vi "ALLPROPS0dll.vi"(8 "error in (no error)":errorcluster, 11 "Inputs":T2) -> (0 "error out":errorcluster, 3 "Outputs":T1)   [LabVIEW 2021]
uses:
  REFPROP.dll
panel:
  # "REFPROP-ALLPROPS0dll.vi"
  # "void ALLPROPS0dll(int *iIn, int *iOut/* 200 */, int *iFlag, double *T, double *D, double *z/* 20 */, double *Output/* 200 */, int *ierr, char *herr, int herr_length/* 255 */);"
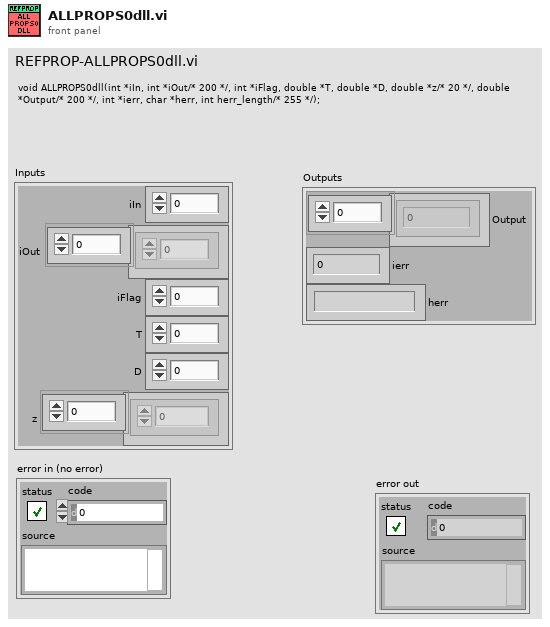
[diagram p1: front panel]
types:
  T1 = cluster{"Output":dbl[], "ierr":i32, "herr":string}
  T2 = cluster{"iIn":i32, "iOut":i32[], "iFlag":i32, "T":dbl, "D":dbl, "z":dbl[]}
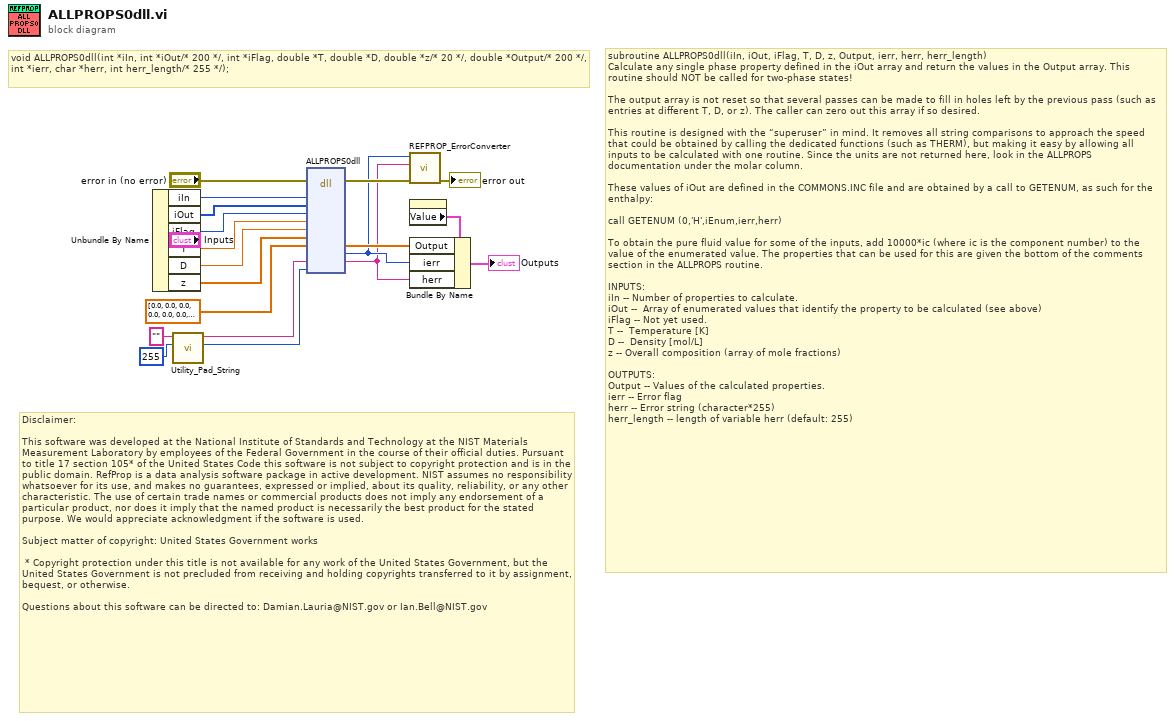
[diagram p0: block diagram]
diagram:
  # "void ALLPROPS0dll(int *iIn, int *iOut/* 200 */, int *iFlag, double *T, double *D, double *z/* 20 */, double *Output/* 200 */, int *ierr, char *herr, int herr_length/* 255 */);"
  # "Disclaimer:\n\nThis software was developed at the National Institute of Standards and Technology at the NIST Materials Measurement Laboratory by employees of the Federal Government in the course of their official duties. Pursuant to title 17 section 105* of the United States Code this software is not subject to copyright protection and is in the public domain. RefProp is a data analysis software package in active development. NIST assumes no responsibility whatsoever for its use, and makes no guarantees, expressed or implied, about its quality, reliability, or any other characteristic. The use of certain trade names or commercial products does not imply any endorsement of a particular product, nor does it imply that the named product is necessarily the best product for the stated purpose. We would appreciate acknowledgment if the software is used.\n \nSubject matter of copyright: United States Government works\n  \n * Copyright protection under this title is not available for any work of the United States Government, but the United States Government is not precluded from receiving and holding copyrights transferred to it by assignment, bequest, or otherwise.\n\nQuestions about this software can be directed to: Damian.Lauria@NIST.gov or Ian.Bell@NIST.gov"
  # "subroutine ALLPROPS0dll(iIn, iOut, iFlag, T, D, z, Output, ierr, herr, herr_length)\nCalculate any single phase property defined in the iOut array and return the values in the Output array. This routine should NOT be called for two-phase states!\n\nThe output array is not reset so that several passes can be made to fill in holes left by the previous pass (such as entries at different T, D, or z). The caller can zero out this array if so desired.\n\nThis routine is designed with the “superuser” in mind. It removes all string comparisons to approach the speed that could be obtained by calling the dedicated functions (such as THERM), but making it easy by allowing all inputs to be calculated with one routine. Since the units are not returned here, look in the ALLPROPS documentation under the molar column.\n\nThese values of iOut are defined in the COMMONS.INC file and are obtained by a call to GETENUM, as such for the enthalpy:\n\ncall GETENUM (0,'H',iEnum,ierr,herr)\n\nTo obtain the pure fluid value for some of the inputs, add 10000*ic (where ic is the component number) to the value of the enumerated value. The properties that can be used for this are given the bottom of the comments section in the ALLPROPS routine.\n\nINPUTS:\t\niIn -- Number of properties to calculate.\niOut --  Array of enumerated values that identify the property to be calculated (see above)\niFlag -- Not yet used.\nT --  Temperature [K]\nD --  Density [mol/L]\nz -- Overall composition (array of mole fractions)\n\nOUTPUTS:\nOutput -- Values of the calculated properties.\nierr -- Error flag\nherr -- Error string (character*255)\nherr_length -- length of variable herr (default: 255)"
  n1 = Unbundle By Name("Inputs") -> ("iIn"=w18:i32, "iOut"=w17:i32[], "iFlag"=w16:i32, "T"=w15:dbl, "D"=w14:dbl, "z"=w13:dbl[])
  n2 = call "Utility_Pad_String.vi"("Target Length"=255, "String in"="") -> ("Length out"=w1:i32, "result string"=w2:string)  [unwired: 7 in, 1 out]
  n3 = dll-call lib="C:/Users/lauria/OneDrive - NIST/LabVIEW Projects/7 REFPROP/REFPROP-wrappers-master/REFPROP-wrappers-master/wrappers/LabVIEW/REFPROP/REFPROP.dll" fn="ALLPROPS0dll"(error in="error in (no error)", "iIn"=w18, "iOut"=w17, "iFlag"=w16, "T"=w15, "D"=w14, "z"=w13, "Output"=dbl[] [0.0, 0.0, 0.0, 0.0, 0.0, 0.0, 0.0, 0.0, 0.0, 0.0, 0.0, 0.0, 0.0, 0.0, 0.0, 0.0, 0.0, 0.0, 0.0, 0.0, 0.0, 0.0, 0.0, 0.0, 0.0, 0.0, 0.0, 0.0, 0.0, 0.0, 0.0, 0.0, 0.0, 0.0, 0.0, 0.0, 0.0, 0.0, 0.0, 0.0, 0.0, 0.0, 0.0, 0.0, 0.0, 0.0, 0.0, 0.0, 0.0, 0.0, 0.0, 0.0, 0.0, 0.0, 0.0, 0.0, 0.0, 0.0, 0.0, 0.0, 0.0, 0.0, 0.0, 0.0, 0.0, 0.0, 0.0, 0.0, 0.0, 0.0, 0.0, 0.0, 0.0, 0.0, 0.0, 0.0, 0.0, 0.0, 0.0, 0.0, 0.0, 0.0, 0.0, 0.0, 0.0, 0.0, 0.0, 0.0, 0.0, 0.0, 0.0, 0.0, 0.0, 0.0, 0.0, 0.0, 0.0, 0.0, 0.0, 0.0, 0.0, 0.0, 0.0, 0.0, 0.0, 0.0, 0.0, 0.0, 0.0, 0.0, 0.0, 0.0, 0.0, 0.0, 0.0, 0.0, 0.0, 0.0, 0.0, 0.0, 0.0, 0.0, 0.0, 0.0, 0.0, 0.0, 0.0, 0.0, 0.0, 0.0, 0.0, 0.0, 0.0, 0.0, 0.0, 0.0, 0.0, 0.0, 0.0, 0.0, 0.0, 0.0, 0.0, 0.0, 0.0, 0.0, 0.0, 0.0, 0.0, 0.0, 0.0, 0.0, 0.0, 0.0, 0.0, 0.0, 0.0, 0.0, 0.0, 0.0, 0.0, 0.0, 0.0, 0.0, 0.0, 0.0, 0.0, 0.0, 0.0, 0.0, 0.0, 0.0, 0.0, 0.0, 0.0, 0.0, 0.0, 0.0, 0.0, 0.0, 0.0, 0.0, 0.0, 0.0, 0.0, 0.0, 0.0, 0.0, 0.0, 0.0, 0.0, 0.0, 0.0, 0.0, 0.0, 0.0, 0.0, 0.0, 0.0, 0.0], "herr"=w2, "herr_length"=w1) -> (error out=w11:errorcluster, "Output"=w7:dbl[], "ierr"=w6:i32, "herr"=w5:string)  [unwired: 11 in, 1 out]
  n4 = call "REFPROP_ErrorConverter.vi"("error in (no error)"=w11, "Error Message"=w5, "Error Code"=w6) -> ("error out"=→"error out":errorcluster)  [unwired: 8 in]
  n5 = property on="Outputs" class="Clust (strict)"() -> ("Value"=w8:T1)  [unwired: 2 in, 2 out]
  n6 = Bundle By Name(cluster=w8, "Output"=w7, "ierr"=w6, "herr"=w5) -> (→"Outputs":T1)
